vi "archivotxtescritura.vi"() -> ()   [LabVIEW 2016]
panel:
  in  "file path (use dialog)":path
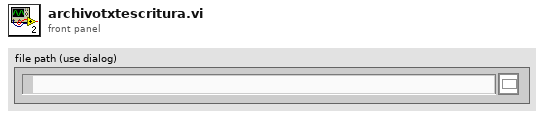
[diagram p1: front panel]
types:
  T1 = enum16{"open", "replace", "create", "open or create", "replace or create", "replace or create with confirmation"}
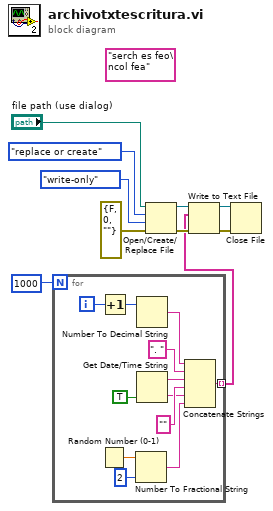
[diagram p0: block diagram]
diagram:
  (unwired) "serch es feo\ncol fea" ("text")
  n1 = for {
    N: 1000 -> [_]
    tunnel: [w13] -> w1 mode=indexing
    i -> [w22]
    n2 = Random Number (0-1)() -> (number: 0 to 1=w20:dbl)
    n3 = Increment(x=w22) -> (x+1=w21:i32)
    n4 = Number To Fractional String(number=w20, precision (6)=i16 2) -> (F-format string=w14:string)  [unwired: 2 in]
    n5 = Number To Decimal String(number=w21) -> (decimal integer string=w19:string)  [unwired: 1 in]
    n6 = Get Date/Time String(want seconds? (F)=TRUE) -> (date string=w17:string, time string=w15:string)  [unwired: 2 in]
    n7 = Concatenate Strings(w19, ". ", w17, "", w15, w14) -> (w13:string)
  }
  n8 = Open/Create/Replace File(file path (use dialog)="file path (use dialog)", error in=errorcluster {"status"=FALSE, "code"=0, "source"=""}, operation (0:open)=T1."replace or create", access (0:read/write)=enum16{"read/write", "read-only", "write-only"}."write-only") -> (refnum out=w5:refnum<file>, error out=w6:errorcluster)  [unwired: 2 in, 1 out]
  n9 = Write to Text File(file (use dialog)=w5, text=w1, error in=w6) -> (refnum out=w3:refnum<file>, error out=w4:errorcluster)  [unwired: 1 in, 1 out]
  n10 = Close File(refnum=w3, error in=w4) -> ()  [unwired: 2 out]
